vi "Rysuj percepcje.vi"(4 "color(black)":u32(colorbox), 6 "pen (Width 5)":T1={"Width"=5, "Style"=enum."Solid"}, 7 "Swiat in":picture, 8 "error in (no error)":errorcluster, 11 "Swiat in":refnum<class "Swiat.lvclass">) -> (0 "error out":errorcluster, 3 "Swiat out":refnum<class "Swiat.lvclass">, 5 "Swiat out":picture)   [LabVIEW 2014, in "Swiat.lvclass"]
uses:
  Swiat.lvclass
  Swiat.lvclass/Swiat.ctl
  Boid/Boid.lvclass/Boid.ctl
  Boid/Boid.lvclass
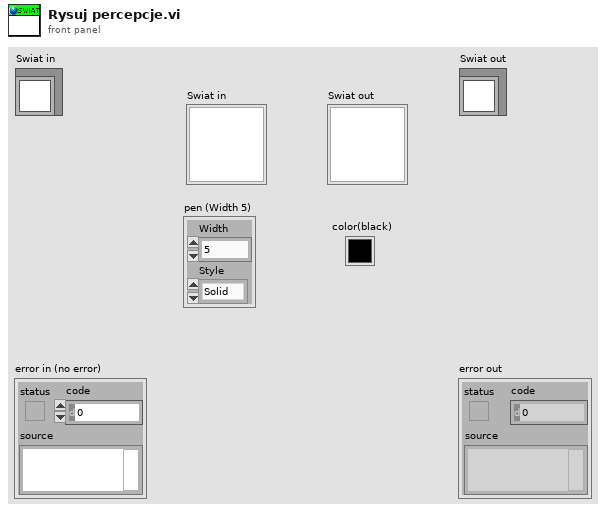
[diagram p1: front panel]
types:
  T1 = cluster{"Width":u16, "Style":enum32{"Solid", "Dash", "Dot", "DashDot", "DashDotDot"}}
  T2 = typedef "Position.ctl" = cluster{"x":i16, "y":i16}
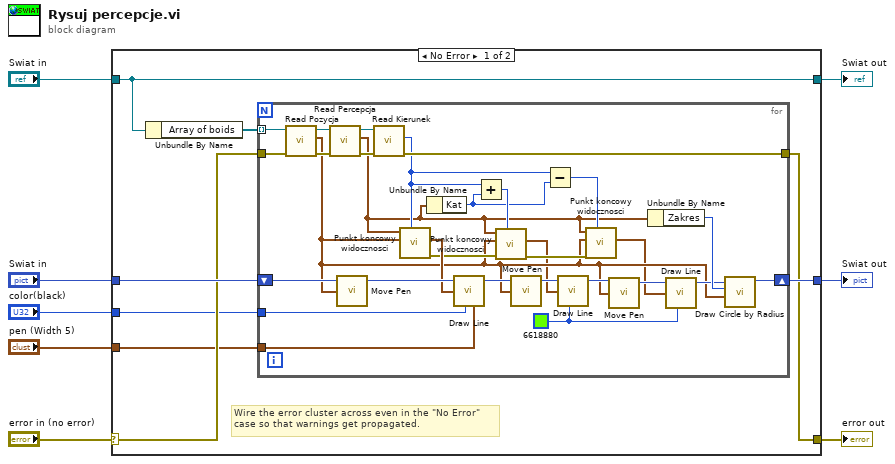
[diagram p0: block diagram]
diagram:
  n1 = case shown="No Error" "error in (no error)" {
    selector: "error in (no error)" -> [w12 w49]
    tunnel: [w11 w49] -> w7
    tunnel: [w16 w48] -> w5
    tunnel: "Swiat in" -> [w16 w48]
    tunnel: "Swiat in" -> [w14 w47]
    tunnel: [w13 w47] -> w3
    tunnel: "pen (Width 5)" -> [w10 _]
    tunnel: "color(black)" -> [w9 _]
    frame No Error {
      # "Wire the error cluster across even in the \"No Error\"\ncase so that warnings get propagated."
      n2 = Unbundle By Name(w16) -> ("Array of boids"=w15:refnum<class "Boid.lvclass">[])
      n3 = for {
        tunnel: w15 -> [w42] mode=indexing
        shift-right: [w35] -> w13
        shift-left: w14 -> [w37]
        tunnel: w12 -> [w40]
        tunnel: [w38] -> w11
        tunnel: w10 -> [w46]
        tunnel: w9 -> [w45]
        w17 = u32 6618880 ("color(black)")
        n4 = call "Read Pozycja.vi"("error in (no error)"=w40, "Boid in"=w42) -> ("error out"=w39:errorcluster, "Position"=w25:T2, "Boid out"=w41:refnum<class "Boid.lvclass">)  [unwired: 7 in]
        n5 = call "Read Percepcja.vi"("error in (no error)"=w39, "Boid in"=w41) -> ("error out"=w43:errorcluster, "Percepcja"=w19:cluster{"Zakres":i16, "Kat":i16}, "Boid out"=w44:refnum<class "Boid.lvclass">)  [unwired: 7 in]
        n6 = call <vilib>:"Move Pen.vi"("new position"=w25, "picture"=w37) -> ("new picture"=w36:picture)  [unwired: 3 in]
        n7 = call "Read Kierunek.vi"("error in (no error)"=w43, "Boid in"=w44) -> ("error out"=w38:errorcluster, "Kierunek"=w22:i16)  [unwired: 7 in, 1 out]
        n8 = call "Punkt koncowy widocznosci.vi"("Kierunek"=w22, "Start Pos"=w25, "Percepcja"=w19) -> ("error out"=w27:errorcluster, "Final Pos"=w34:T2)  [unwired: 7 in]
        n9 = Unbundle By Name(w19) -> ("Kat"=w18:i16)
        n10 = call <vilib>:"Draw Line.vi"("picture"=w36, "end point"=w34, "color(black)"=w45, "pen"=w46) -> ("new picture"=w32:picture)  [unwired: 5 in]
        n11 = Add(x=w22, y=w18) -> (x+y=w21:i16)
        n12 = call "Punkt koncowy widocznosci.vi"("Kierunek"=w21, "error in (no error)"=w27, "Start Pos"=w25, "Percepcja"=w19) -> ("error out"=w26:errorcluster, "Final Pos"=w23:T2)  [unwired: 6 in]
        n13 = call <vilib>:"Move Pen.vi"("new position"=w25, "picture"=w32) -> ("new picture"=w31:picture)  [unwired: 3 in]
        n14 = Subtract(x=w22, y=w18) -> (x-y=w20:i16)
        n15 = call <vilib>:"Draw Line.vi"("picture"=w31, "end point"=w23, "color(black)"=w17) -> ("new picture"=w28:picture)  [unwired: 6 in]
        n16 = call "Punkt koncowy widocznosci.vi"("Kierunek"=w20, "error in (no error)"=w26, "Start Pos"=w25, "Percepcja"=w19) -> ("Final Pos"=w24:T2)  [unwired: 6 in, 1 out]
        n17 = call <vilib>:"Move Pen.vi"("new position"=w25, "picture"=w28) -> ("new picture"=w30:picture)  [unwired: 3 in]
        n18 = Unbundle By Name(w19) -> ("Zakres"=w33:i16)
        n19 = call <vilib>:"Draw Line.vi"("picture"=w30, "end point"=w24, "color(black)"=w17) -> ("new picture"=w29:picture)  [unwired: 6 in]
        n20 = call <vilib>:"Draw Circle by Radius.vi"("pixel center"=w25, "radius"=w33, "picture"=w29) -> ("new picture"=w35:picture)  [unwired: 8 in]
      }
    }
    frame Error {
    }
  }
  "error out" <- w7
  "Swiat out" <- w5
  "Swiat out" <- w3
